vi "group Bulk Read Tx Rx Packet.vi"(11 "group_num":i32) -> ()   [LabVIEW 2016, in "dxl_x86_c.lvlib"]
doc: "WINDECLSPEC void groupBulkReadTxRxPacket (int group_num);"
uses:
  dxl_x86_c.lvlib
  dxl_x86_c.dll
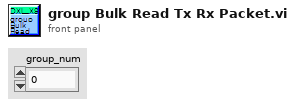
[diagram p1: front panel]
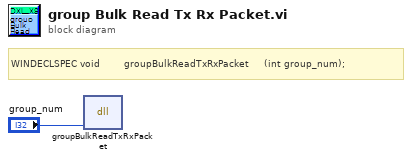
[diagram p0: block diagram]
diagram:
  # "WINDECLSPEC void        groupBulkReadTxRxPacket     (int group_num);"
  n1 = dll-call lib="C:/Users/Platform/Desktop/GITHUB/DynamixelSDK/labview/dxl_x86_c.lvlib/dxl_x86_c.*" fn="groupBulkReadTxRxPacket"("group_num"="group_num") -> ()  [unwired: 5 in, 2 out]
